vi "Read U8 Array.vi"(8 "error in":errorcluster, 9 "size":i32, 10 "register name":string, 11 "session in":u32) -> (0 "error out":errorcluster, 2 "Value out":u8[](array[numeric]), 3 "session out":u32)   [LabVIEW 2018, in "Scalar IO Operations.lvlib"]
uses:
  Scalar IO Operations.lvlib
  NiFpga.dll
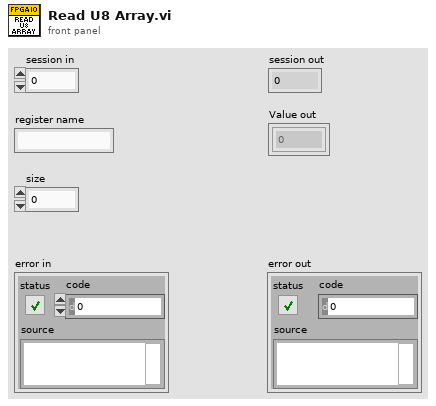
[diagram p1: front panel]
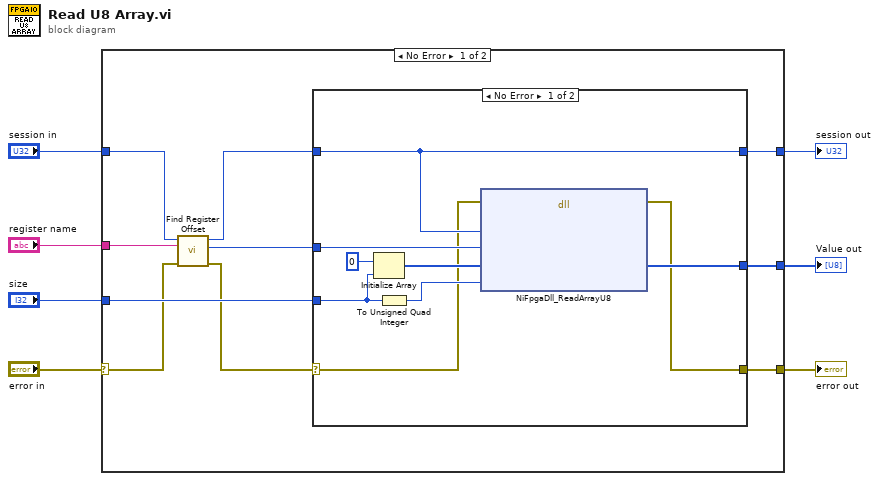
[diagram p0: block diagram]
diagram:
  n1 = case shown="No Error" "error in" {
    selector: "error in" -> [w9 w29]
    tunnel: [w17 w29] -> w7
    tunnel: [w16 w30] -> w6
    tunnel: "size" -> [w15 _]
    tunnel: [w14 _] -> w4
    tunnel: "session in" -> [w13 w30]
    tunnel: "register name" -> [w8 _]
    frame No Error {
      n2 = call "Find Register Offset.vi"("error in (no error)"=w9, "register name"=w8, "session in"=w13) -> ("error out"=w10:errorcluster, "resource offset"=w11:u32, "session out"=w12:u32)  [unwired: 6 in]
      n3 = case shown="No Error" w10 {
        selector: w10 -> [w19 w28]
        tunnel: w12 -> [w23 w27]
        tunnel: [w18 w28] -> w17
        tunnel: w11 -> [w22 _]
        tunnel: [w23 w27] -> w16
        tunnel: w15 -> [w21 _]
        tunnel: [w20 _] -> w14
        frame No Error {
          n4 = Initialize Array(u8 0, w21) -> (w25:u8[])
          n5 = To Unsigned Quad Integer(1:w21) -> (0:w26:u64)
          n6 = dll-call lib="NiFpga.*" fn="NiFpgaDll_ReadArrayU8"(error in=w19, "session"=w23, "offset"=w22, "data"=w25, "count"=w26) -> (error out=w18:errorcluster, "data"=w20:u8[])  [unwired: 6 in, 1 out]
        }
        frame Error {
        }
      }
    }
    frame Error {
    }
  }
  "error out" <- w7
  "session out" <- w6
  "Value out" <- w4
